vi "JKISM++ State Dashboard - DebugTool.vi"() -> ()   [LabVIEW 2014]
uses:
  _Support/Typedef/_JKISM Current State.ctl
  _Support/GlobalEvent/FGV-GlobalEventRef.vi
  <resource>/dialog/lvconfig.llb/LV Config Write Numeric (I32).vi
  <resource>/dialog/lvconfig.llb/LV Config Read Numeric (I32).vi
  _Support/jkism-tool-support.lvlib
  JKI State Machine++.lvlib
panel:
  in  "Clear JKISM":bool
  out "Dashboard":T1(array[cluster])
  out "State History":string
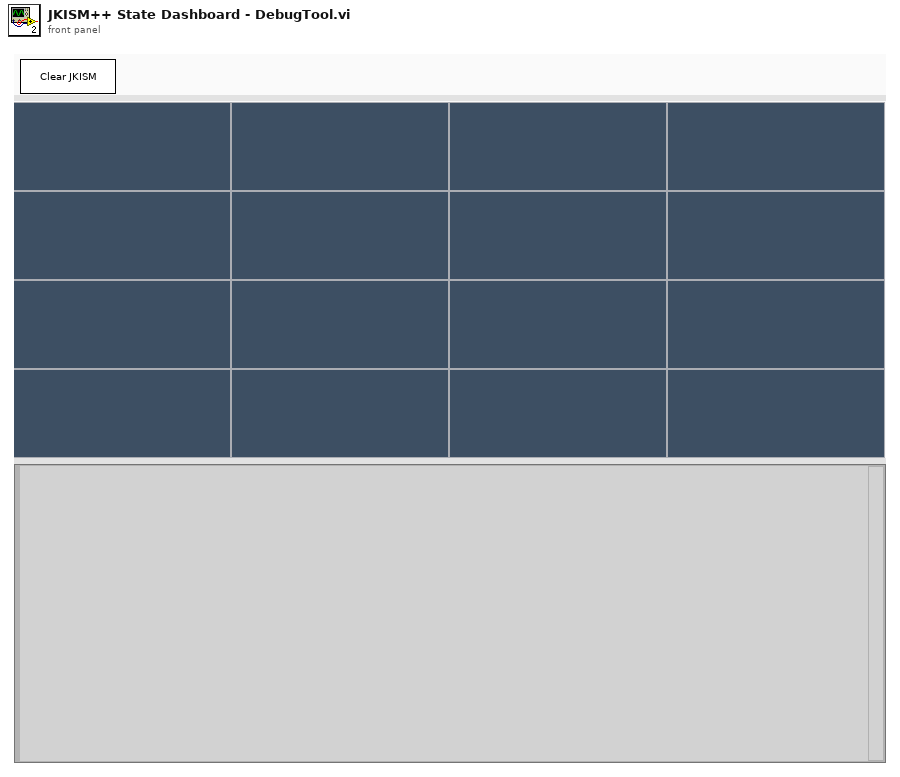
[diagram p1: front panel]
types:
  T1 = cluster{"Label":string, "Value":string, "String":string}[][]
  T2 = enum32{"Invalid", "Standard", "Closed", "Hidden", "Minimized", "Maximized"}
  T3 = enum32{"invalid app kind", "Development System", "Run Time System", "Student Edition", "Embedded LabVIEW", "Evaluation", "Custom"}
  T4 = typedef "JKI State Machine++.lvlib/_JKISM Current State.ctl" = cluster{"Name(\"\" to use uuid)":string, "Current State":string, "Arguments":string, "Argument - State":string, "From Who":string, "Complete(T)/Start(F)":bool}
  T5 = cluster{"Label":string, "Value":string, "String":string}
  T6 = cluster{"Core":cluster{"Current VI Reference":refnum<vi>, "Close Panel on Exit?":bool}, "Global-DataTable":string[][], "NumCols":i16, "NumRows":i16, "JKISM Global Log Event":refnum<user-event>, "Log":T4}
  T7 = cluster{"Current VI Reference":refnum<vi>, "Close Panel on Exit?":bool}
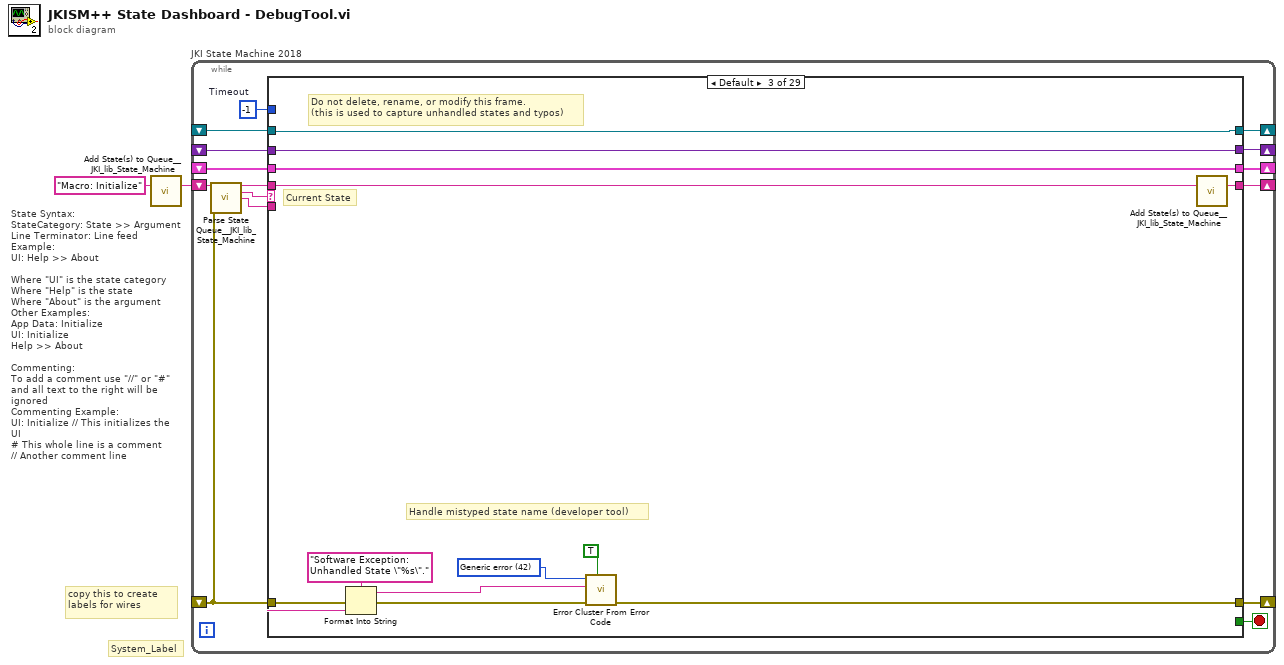
[diagram p0: block diagram]
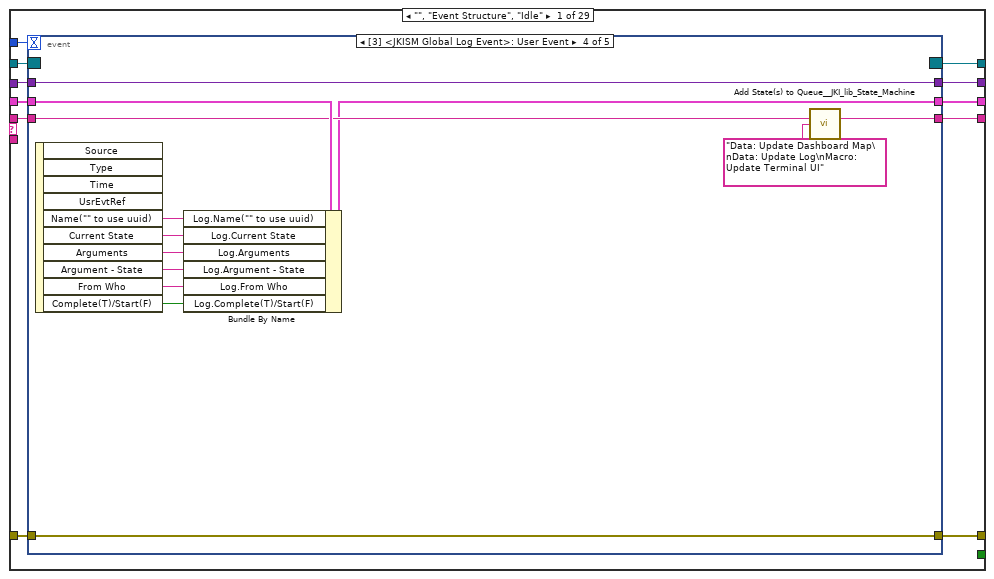
[diagram p2: hidden frame]
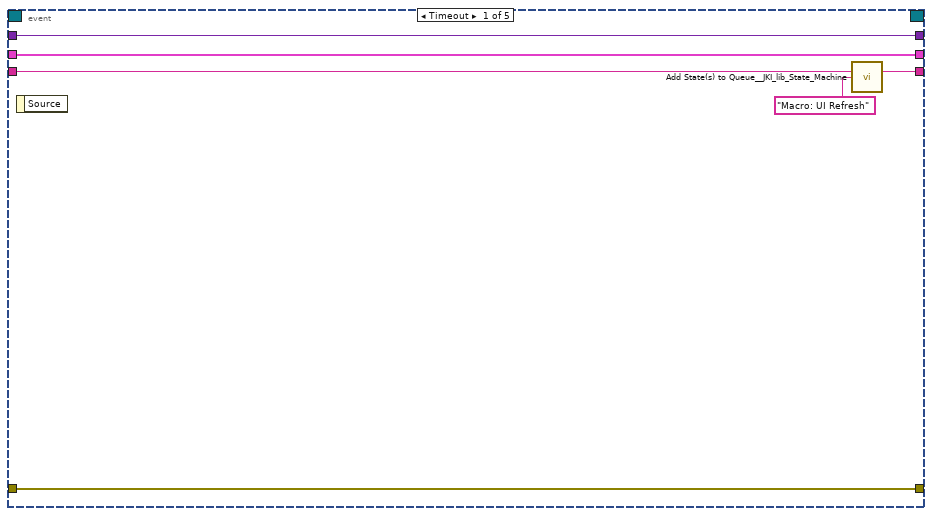
[diagram p3: hidden frame]
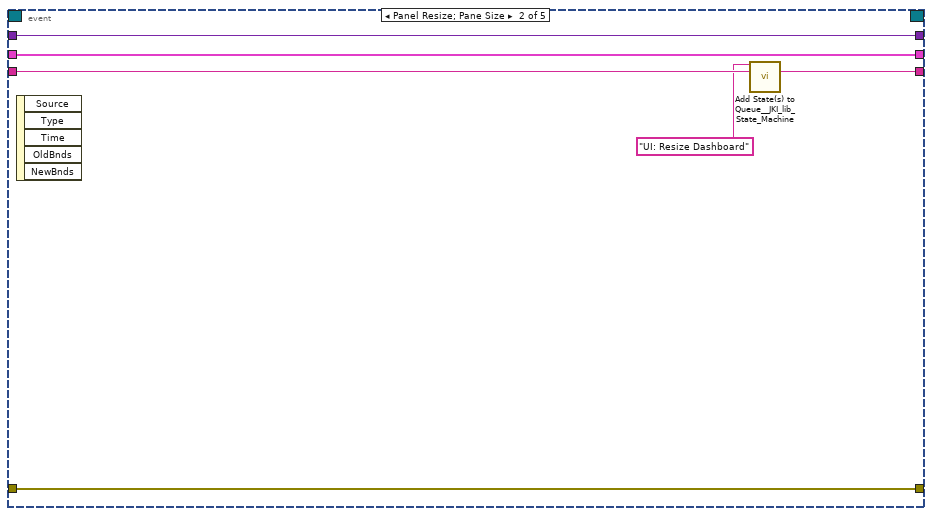
[diagram p4: hidden frame]
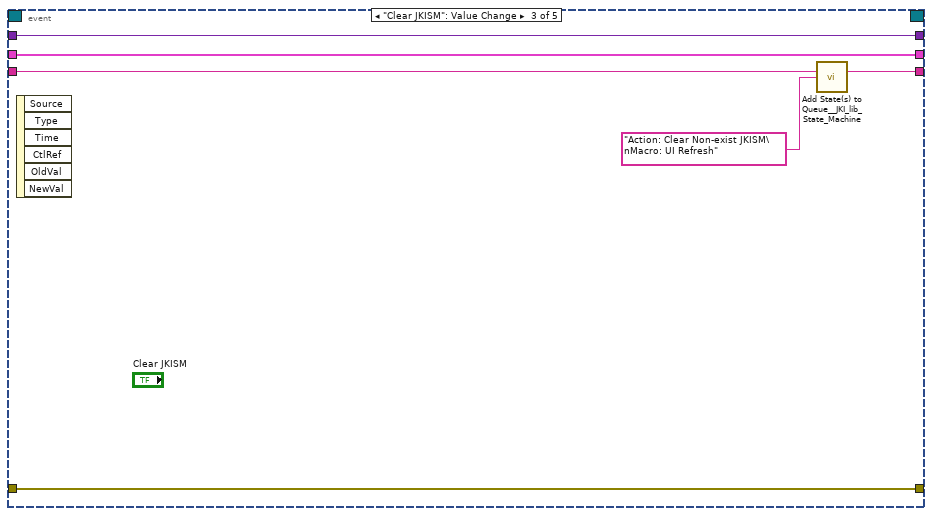
[diagram p5: hidden frame]
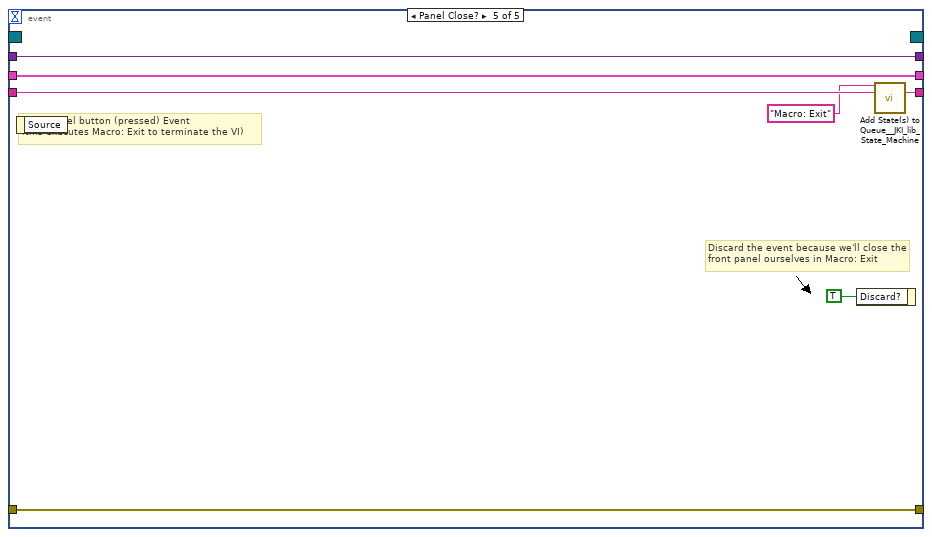
[diagram p6: hidden frame]
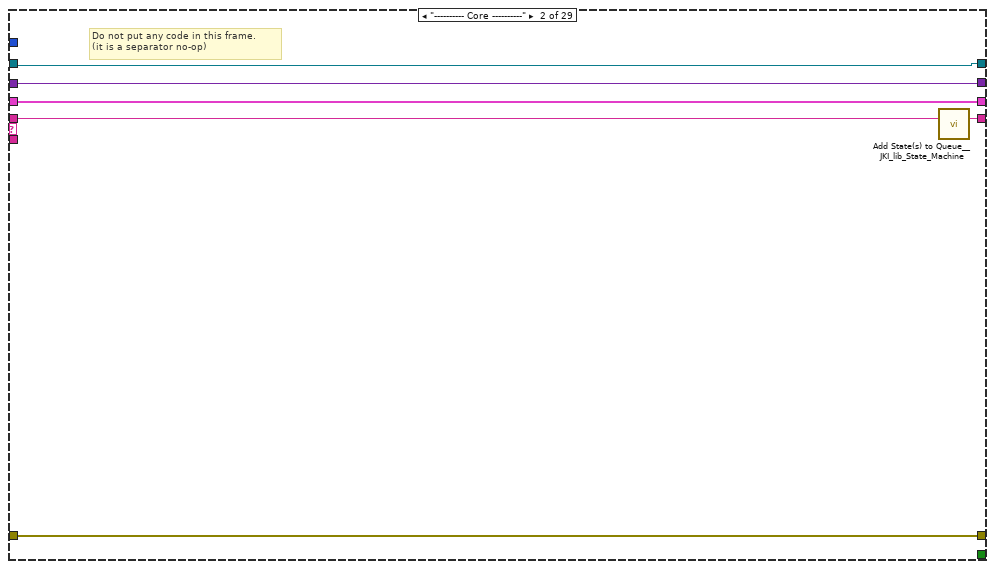
[diagram p7: hidden frame]
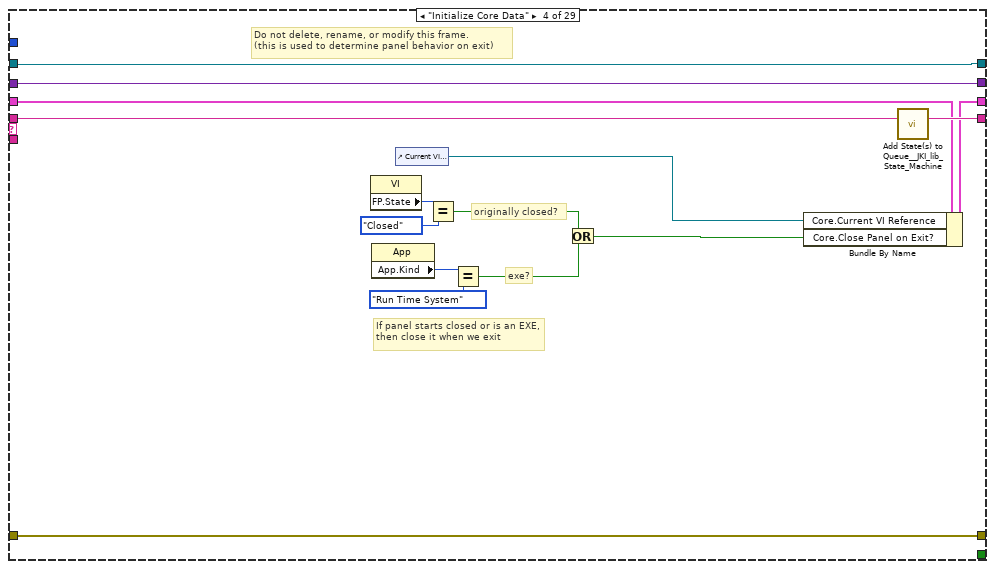
[diagram p8: hidden frame]
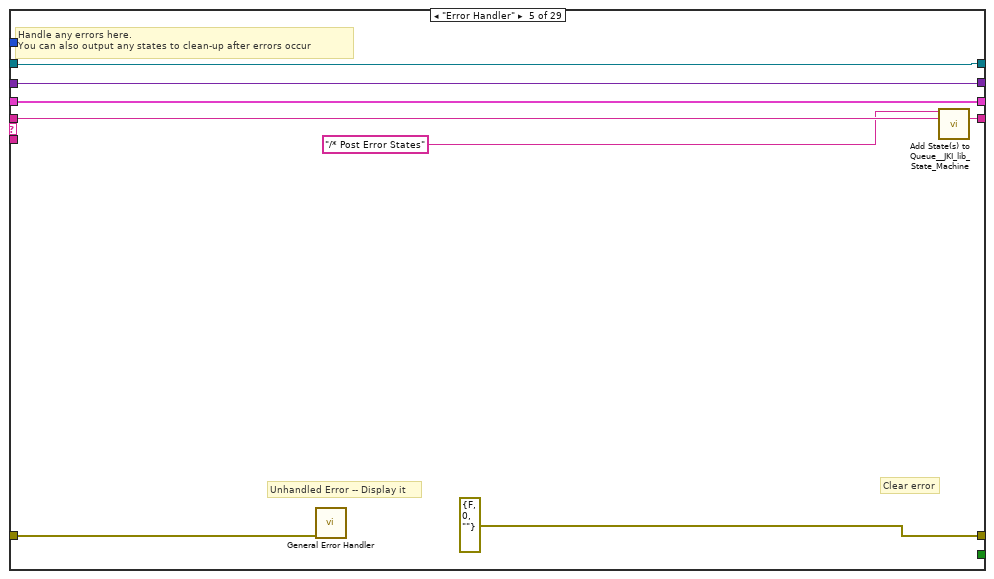
[diagram p9: hidden frame]
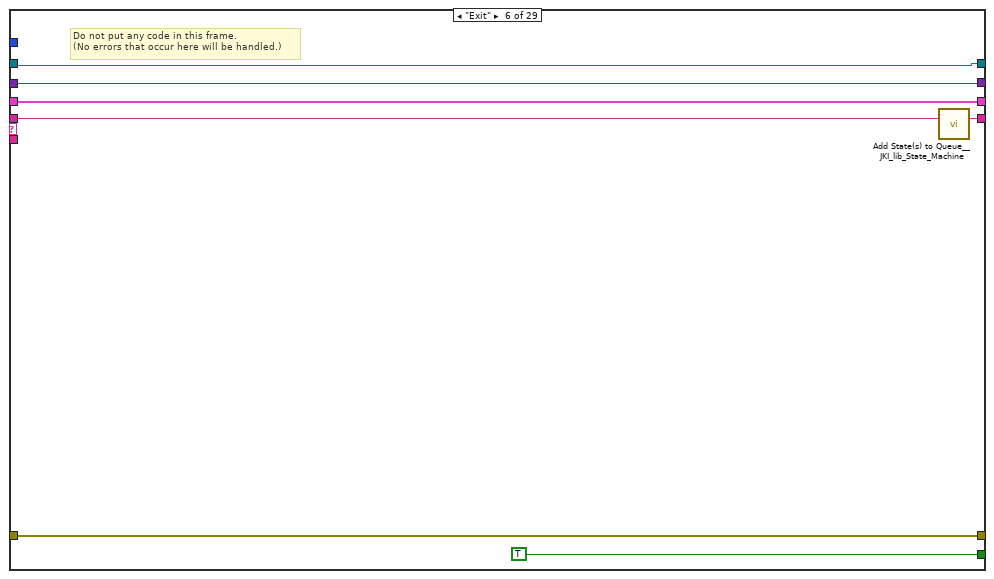
[diagram p10: hidden frame]
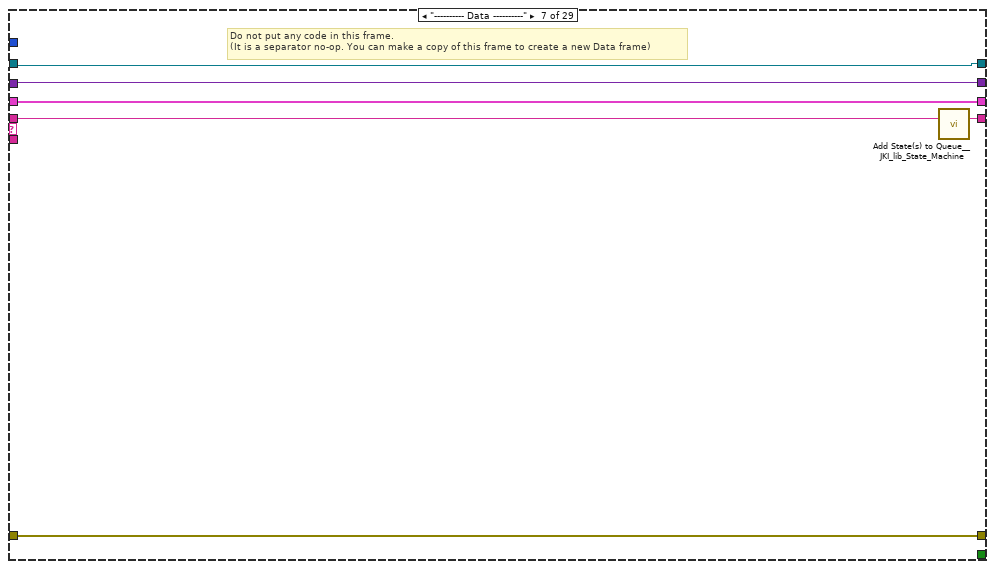
[diagram p11: hidden frame]
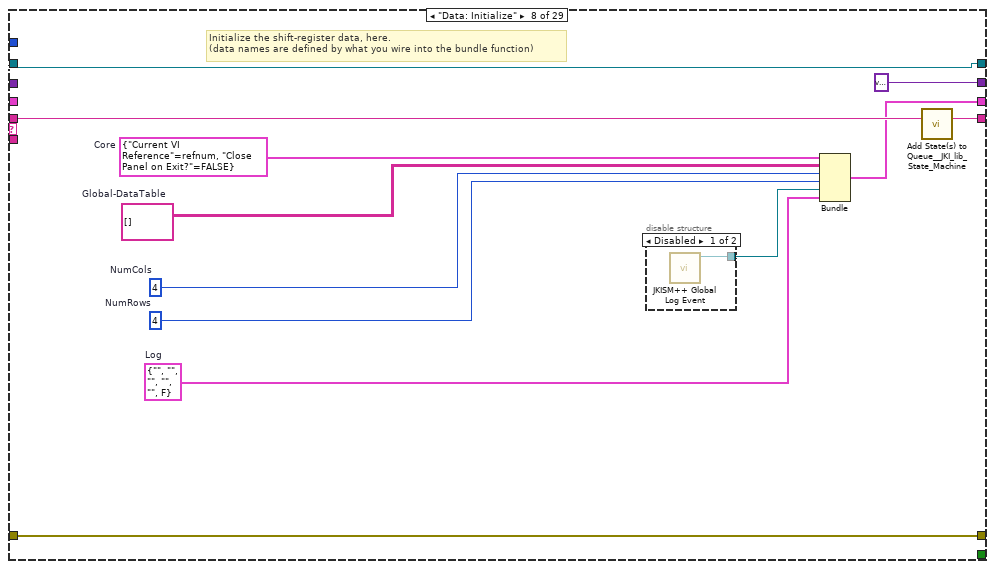
[diagram p12: hidden frame]
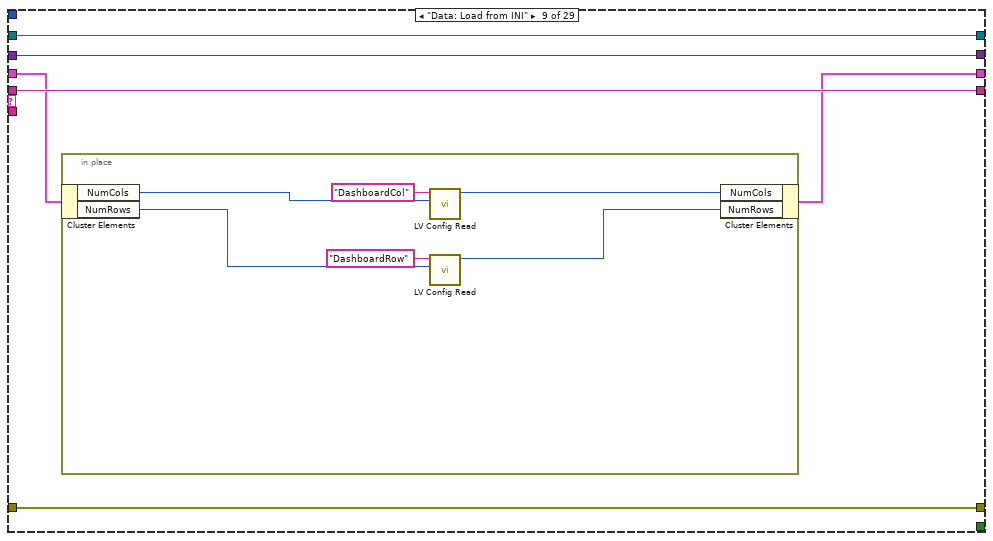
[diagram p14: hidden frame]
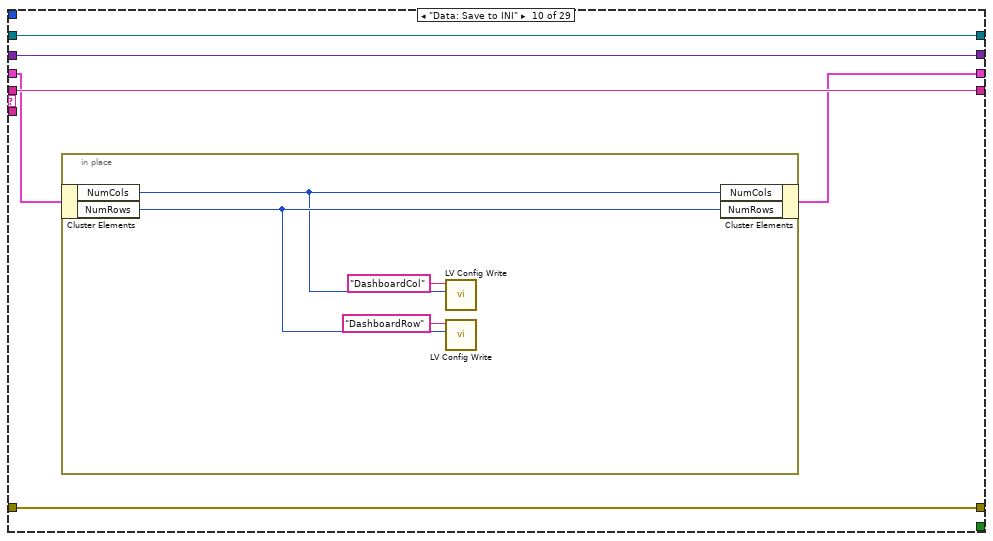
[diagram p15: hidden frame]
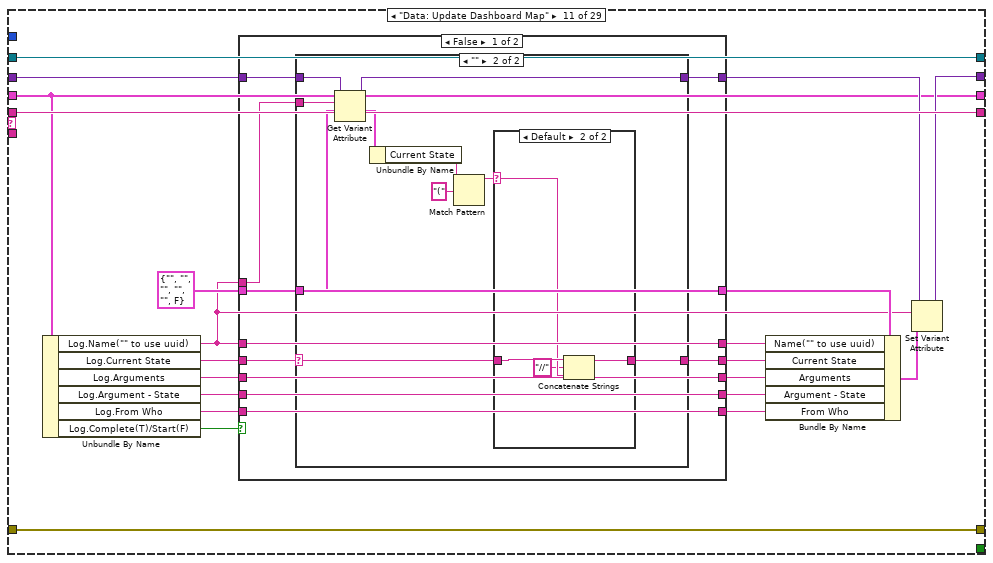
[diagram p16: hidden frame]
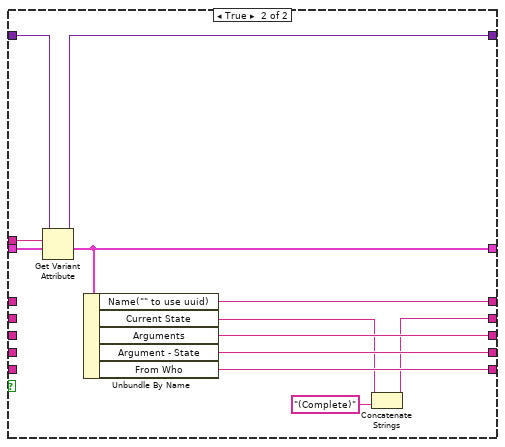
[diagram p19: hidden frame]
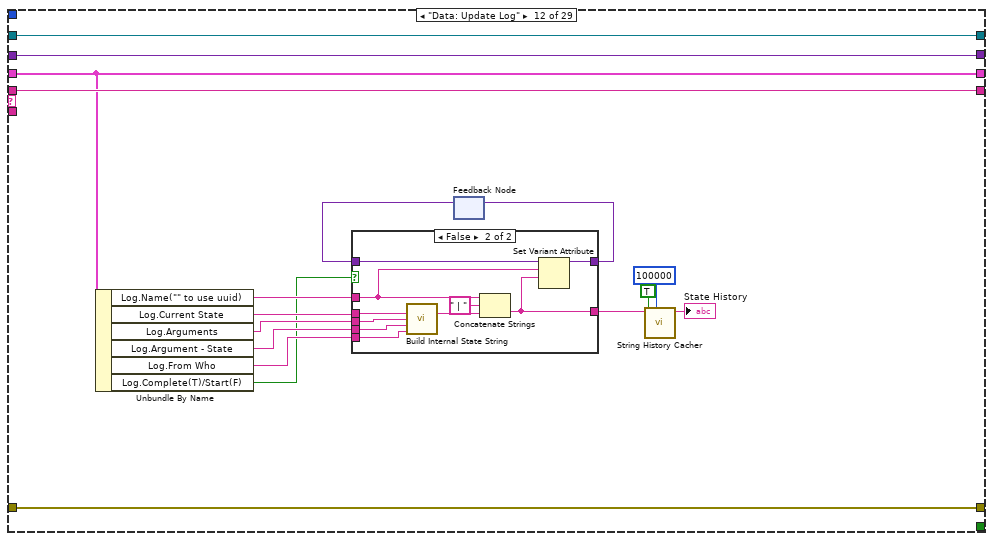
[diagram p20: hidden frame]
diagram:
  # "State Syntax:\nStateCategory: State >> Argument\nLine Terminator: Line feed\nExample:\nUI: Help >> About\n\nWhere \"UI\" is the state category\nWhere \"Help\" is the state\nWhere \"About\" is the argument\nOther Examples:\nApp Data: Initialize\nUI: Initialize\nHelp >> About\n\nCommenting:\nTo add a comment use \"//\" or \"#\" and all text to the right will be ignored\nCommenting Example:\nUI: Initialize // This initializes the UI\n# This whole line is a comment\n// Another comment line"
  # "copy this to create labels for wires"
  # "System_Label"
  n1 = call <vilib>:"Add State(s) to Queue__JKI_lib_State_Machine.vi"("State(s) in (\"\")"="Macro: Initialize") -> ("States Out"=w1:string)  [unwired: 14 in]
  n2 = while "JKI State Machine 2018" {
    shift-right: [w10] -> _
    shift-left: _ -> [w9]
    shift-right: [w13] -> _
    shift-left: _ -> [w7]
    shift-right: [w12] -> _
    shift-left: w1 -> [w14]
    shift-right: [w6] -> _
    shift-left: _ -> [w5]
    shift-right: [w4] -> _
    shift-left: _ -> [w3]
    stop <- w11 stop-if-true
    w8 = -1  # Timeout
    n3 = call <vilib>:"Parse State Queue__JKI_lib_State_Machine.vi"("State Queue"=w14, "Error In (no error)"=w7) -> ("Remaining States"=w16:string, "Current State"=w17:string, "Arguments"=w15:string)  [unwired: 11 in]
    n4 = case shown="Default" w17 {
      selector: w17 -> [_ _ w75 _ _ _ _ _ _ _ _ _ _ _ _ _ _ _ _ _ _ _ _ _ _ _ _ _ _]
      tunnel: w16 -> [w28 w72 w79 w100 w108 w115 w121 w133 w139 w151 w176 w232 w259 w265 w274 w286 w299 w376 w391 w401 w409 w417 w424 w431 w439 w446 w459 w463 w474]
      tunnel: w15 -> [_ _ _ _ _ _ _ _ _ _ _ _ _ _ _ w281 w293 _ _ _ _ _ _ _ _ _ _ _ _]
      tunnel: w9 -> [w26 w69 w77 w93 w105 w113 w118 _ w138 w150 w163 w223 w254 w262 w270 w284 w295 w372 w388 w400 w408 w413 w421 w428 w434 w443 w456 w462 w473]
      tunnel: [w25 w70 w81 w97 errorcluster {"status"=FALSE, "code"=0, "source"=""} ("error out") w112 w119 w129 w140 w152 w177 w233 w253 w263 w272 w282 w296 w373 w389 w402 w410 w418 w422 w429 w437 w444 w457 w464 w475] -> w13
      tunnel: w7 -> [w24 w70 w80 w97 w104 w112 w119 w129 w140 w152 w177 w233 w256 w263 w272 w283 w297 _ w389 w402 w410 w418 w422 w429 w437 w444 w457 w464 w475]
      tunnel: [w27 w71 w78 w99 w107 w114 w120 w132 w139 w151 w176 w232 w258 w264 w273 w285 w298 w375 w390 w401 w409 w417 w423 w430 w438 w445 w458 w463 w474] -> w12
      tunnel: [_ _ _ _ _ TRUE _ _ _ _ _ _ _ _ _ _ _ _ _ _ _ _ _ _ _ _ _ _ _] -> w11
      tunnel: [w23 w69 w77 w98 w105 w113 w118 w131 w137 w149 w163 w223 w254 w262 w270 w284 w295 w372 w388 w400 w404 w413 w421 w428 w434 w443 w456 w462 w473] -> w10
      tunnel: w8 -> [w22 _ _ _ _ _ _ _ _ _ _ _ _ _ _ _ _ _ _ _ _ _ _ _ _ _ _ _ _]
      tunnel: [w20 w68 w74 w87 w102 w110 w117 variant w136 w148 w164 w231 w252 w261 w267 w280 w292 w369 w383 w399 w407 w416 w420 w426 w433 w441 w449 w461 w469] -> w6
      tunnel: w5 -> [w21 w68 w74 w87 w102 w110 w117 _ w136 w148 w165 w231 w252 w261 w267 w280 w292 w369 w382 w399 w407 w416 w420 w426 w433 w441 w449 w461 w471]
      tunnel: [w18 w67 w73 w86 w101 w109 w116 w124 w135 w147 w175 w230 w251 w260 w266 w279 w291 w368 w379 w398 w405 w415 w419 w425 w432 w440 w448 w460 w472] -> w4
      tunnel: w3 -> [w19 w67 w73 w86 w101 w109 w116 w124 w135 w147 w175 w230 w251 w260 w266 w279 w291 w368 w379 w398 _ w415 w419 w425 w432 w440 w448 w460 w472]
      frame "", "Event Structure", "Idle" {
        n5 = event shown="[3] <JKISM Global Log Event>: User Event" {
          selector: w19 -> [_ _ _ _ _]
          dyn-events: [_ _ _ _ _] -> w18
          timeout: w22 -> [_ _ _ _ _]
          tunnel: w28 -> [w34 w37 w43 w54 w66]
          tunnel: [w33 w38 w42 w58 w65] -> w27
          tunnel: w26 -> [w31 w39 w45 w55 w64]
          tunnel: [w32 w40 w46 w59 w61] -> w25
          tunnel: w24 -> [w32 w40 w46 w59 w61]
          tunnel: [w31 w39 w45 w53 w64] -> w23
          tunnel: w21 -> [w29 w35 w44 w56 w60]
          tunnel: [w29 w35 w44 w56 w60] -> w20
          event Timeout {
            n6 = event-data() -> ()  [unwired: 1 in, 1 out]
            n7 = call <vilib>:"Add State(s) to Queue__JKI_lib_State_Machine.vi"("State(s) in (\"\")"=w34, "State(s) at Back (\"\")"="Macro: UI Refresh" ("State(s) in Front (\"\")")) -> ("States Out"=w33:string)  [unwired: 13 in]
          }
          event Panel Resize; Pane Size {
            n8 = event-data() -> ()  [unwired: 1 in, 5 out]
            n9 = call <vilib>:"Add State(s) to Queue__JKI_lib_State_Machine.vi"("State(s) in Front (\"\")"="UI: Resize Dashboard" ("State(s) in Front (\"\")"), "State(s) in (\"\")"=w37) -> ("States Out"=w38:string)  [unwired: 13 in]
          }
          event "Clear JKISM": Value Change {
            n10 = event-data() -> ()  [unwired: 1 in, 6 out]
            n11 = call <vilib>:"Add State(s) to Queue__JKI_lib_State_Machine.vi"("State(s) in (\"\")"=w43, "State(s) at Back (\"\")"="Action: Clear Non-exist JKISM\nMacro: UI Refresh" ("State(s) at Back (\"\")")) -> ("States Out"=w42:string)  [unwired: 13 in]
          }
          event User Event {
            n12 = event-data() -> ("Name(\"\" to use uuid)"=w47:string, "Current State"=w48:string, "Arguments"=w49:string, "Argument - State"=w50:string, "From Who"=w51:string, "Complete(T)/Start(F)"=w52:bool)  [unwired: 1 in, 4 out]
            n13 = Bundle By Name(cluster=w55, "Log.Name(\"\" to use uuid)"=w47, "Log.Current State"=w48, "Log.Arguments"=w49, "Log.Argument - State"=w50, "Log.From Who"=w51, "Log.Complete(T)/Start(F)"=w52) -> (w53:T6)
            n14 = call <vilib>:"Add State(s) to Queue__JKI_lib_State_Machine.vi"("State(s) in (\"\")"=w54, "State(s) at Back (\"\")"="Data: Update Dashboard Map\nData: Update Log\nMacro: Update Terminal UI" ("State(s) at Back (\"\")")) -> ("States Out"=w58:string)  [unwired: 13 in]
          }
          event Panel Close? {
            # "Discard the event because we'll close the front panel ourselves in Macro: Exit"
            # "Close Panel button (pressed) Event\n(this executes Macro: Exit to terminate the VI)"
            n15 = event-data() -> ()  [unwired: 1 in, 1 out]
            n16 = event-data("Discard?"=TRUE) -> ()  [unwired: 1 in, 1 out]
            n17 = call <vilib>:"Add State(s) to Queue__JKI_lib_State_Machine.vi"("State(s) in Front (\"\")"="Macro: Exit", "State(s) in (\"\")"=w66) -> ("States Out"=w65:string)  [unwired: 13 in]
          }
        }
      }
      frame "---------- Core ----------" {
        # "Do not put any code in this frame.\n(it is a separator no-op)"
        n18 = call <vilib>:"Add State(s) to Queue__JKI_lib_State_Machine.vi"("State(s) in (\"\")"=w72) -> ("States Out"=w71:string)  [unwired: 14 in]
      }
      frame Default {
        w84 = 42 items=["No error", "Argument error", "Memory is full", "Out of zone", "End of file", "File already open", "Generic file I/O error", "File not found", "File permission error", "Disk is full", "Duplicate path", "Too many files open", "System feature not enabled", "Resource file not found", "Cannot add resource", "Resource not found", "Image not found", "Image memory error", "Pen does not exist", "Config type invalid", "Config token not found", "Config parse error", "Config memory error", "Bad external code format", "Bad external code offset", "External code not present", "Null window", "Destroy window error", "Null menu", "Print aborted", "Bad print record", "Print driver error", "Windows error during printing", "Memory error during printing", "Print dialog error", "Generic print error", "Invalid device refnum", "Device not found", "Device parameter error", "Device unit error", "Cannot open device", "Device call aborted", "Generic error", "Cancelled by user", "Object ID too low", "Object ID too high", "Object not in heap", "Unknown heap", "Unknown object (invalid DefProc)", "Unknown object (DefProc not in table)", "Message out of range", "Invalid (null) method", "Unknown message", "Manager call not supported", "Bad address", "Network operation in progress", "Network operation timed out", "Connection is busy", "Network attribute not supported", "Network error", "Address in use", "System out of memory", "Connection aborted", "Connection refused", "Not connected", "Already connected", "Connection closed", "Initialization error (interapplication manager)", "Bad occurrence", "Wait on unbound occurrence handler", "Occurrence queue overflow", "Datalog type conflict", "Unused", "Unrecognized type (interapplication manager)", "Memory corrupt", "Failed to make temporary DLL", "Old CIN version", "Drag socket not found", "Failed to load drop-object", "Failed to register OLE object", "Failed to release OLE object", "Format specifier type mismatch", "Unknown format specifier", "Too few format specifiers", "Too many format specifiers", "Scan failed", "Newer CIN version", "Error converting to variant", "Runtime menu error", "Password tampered", "Variant attribute not found", "Incompatible variant data type", "Event data is not available", "Event Store is not present", "Occurrence is not found", "Event Queue is not created", "Event info is not available", "Refnum passed is NULL", "Error retrieving Class GUID", "Error retrieving CoClass GUID", "Error retrieving TypeLib GUID.", "Bad built application magic bytes.", "Specific driver is different from the specific driver associated with the Logical Name.", "There is no session opened to the class driver.", "Max Error", "MAX - Error with config objects", "MAX - Error loading configuration", "MAX - Group not supported"]
        # "Current State"
        # "Do not delete, rename, or modify this frame.\n(this is used to capture unhandled states and typos)"
        # "Handle mistyped state name (developer tool)"
        n19 = Format Into String(format string="Software Exception: Unhandled State \"%s\"." ("message"), error in=w80, w75) -> (resulting string=w83:string, error out=w82:errorcluster)  [unwired: 1 in]
        n20 = call <vilib>:"Error Cluster From Error Code.vi"("show call chain? (False)"=TRUE, "error in (no error)"=w82, "error message (\"\")"=w83, "error code (0)"=w84) -> ("error out"=w81:errorcluster)  [unwired: 5 in]
        n21 = call <vilib>:"Add State(s) to Queue__JKI_lib_State_Machine.vi"("State(s) in (\"\")"=w79) -> ("States Out"=w78:string)  [unwired: 14 in]
      }
      frame "Initialize Core Data" {
        # "Do not delete, rename, or modify this frame.\n(this is used to determine panel behavior on exit)"
        # "originally closed?"
        # "exe?"
        # "If panel starts closed or is an EXE, then close it when we exit"
        n22 = property class="VI"() -> ("FP.State"=w90:T2)  [unwired: 2 in, 2 out]
        n23 = property class="App"() -> ("App.Kind"=w96:T3)  [unwired: 2 in, 2 out]
        n24 = control-ref of="Current VI Reference"() -> (w91:refnum<vi>)
        n25 = Equal?(x=w90, y=T2."Closed" ("Front Panel Window:State")) -> (x = y?=w88:bool)
        n26 = Equal?(x=w96, y=T3."Run Time System" ("Application:Kind")) -> (x = y?=w94:bool)
        n27 = Or(x=w88, y=w94) -> (x .or. y?=w92:bool)
        n28 = Bundle By Name(cluster=w93, "Core.Current VI Reference"=w91, "Core.Close Panel on Exit?"=w92) -> (w98:T6)
        n29 = call <vilib>:"Add State(s) to Queue__JKI_lib_State_Machine.vi"("State(s) in (\"\")"=w100) -> ("States Out"=w99:string)  [unwired: 14 in]
      }
      frame "Error Handler" {
        # "Unhandled Error -- Display it"
        # "Handle any errors here.\nYou can also output any states to clean-up after errors occur"
        # "Clear error"
        n30 = call <vilib>:"General Error Handler.vi"("error in (no error)"=w104) -> ()  [unwired: 10 in, 5 out]
        n31 = call <vilib>:"Add State(s) to Queue__JKI_lib_State_Machine.vi"("State(s) in Front (\"\")"="/* Post Error States", "State(s) in (\"\")"=w108) -> ("States Out"=w107:string)  [unwired: 13 in]
      }
      frame "Exit" {
        # "Do not put any code in this frame.\n(No errors that occur here will be handled.)"
        n32 = call <vilib>:"Add State(s) to Queue__JKI_lib_State_Machine.vi"("State(s) in (\"\")"=w115) -> ("States Out"=w114:string)  [unwired: 14 in]
      }
      frame "---------- Data ----------" {
        # "Do not put any code in this frame.\n(It is a separator no-op. You can make a copy of this frame to create a new Data frame)"
        n33 = call <vilib>:"Add State(s) to Queue__JKI_lib_State_Machine.vi"("State(s) in (\"\")"=w121) -> ("States Out"=w120:string)  [unwired: 14 in]
      }
      frame "Data: Initialize" {
        w122 = T4 {"Name(\"\" to use uuid)"="", "Current State"="", "Arguments"="", "Argument - State"="", "From Who"="", "Complete(T)/Start(F)"=FALSE}  # Log
        w127 = i16 4  # NumCols
        w126 = i16 4  # NumRows
        w128 = string[][] []  # Global-DataTable
        w130 = T7 {"Current VI Reference"=refnum, "Close Panel on Exit?"=FALSE}  # Core
        # "Initialize the shift-register data, here.\n(data names are defined by what you wire into the bundle function)"
        n34 = disable-structure shown="Disabled" {
          disable-tunnel: [w134 _] -> w123
          frame Disabled {
            n35 = call "JKISM++ Global Log Event.vi"() -> ("JKISM Global Log Event"=w134:refnum<user-event>)  [unwired: 10 in, 1 out]
          }
          frame Enabled {
          }
        }
        n36 = Bundle("Core"=w130, "Global-DataTable"=w128, "NumCols"=w127, "NumRows"=w126, "JKISM Global Log Event"=w123, "Log"=w122) -> (w131:T6)  [unwired: 1 in]
        n37 = call <vilib>:"Add State(s) to Queue__JKI_lib_State_Machine.vi"("State(s) in (\"\")"=w133) -> ("States Out"=w132:string)  [unwired: 14 in]
      }
      frame "Data: Load from INI" {
        n38 = in-place {
          n39 = in-place-cluster #1(w138) -> ("NumCols"=w142:i16, "NumRows"=w145:i16)
          n40 = call-poly <resource>:"LV Config Read.vi"("default value"=w142, "key"="DashboardCol") -> ("value"=w141:i32)  [unwired: 3 in, 2 out]
          n41 = call-poly <resource>:"LV Config Read.vi"("default value"=w145, "key"="DashboardRow") -> ("value"=w144:i32)  [unwired: 3 in, 2 out]
          n42 = in-place-cluster #1("NumCols"=w141, "NumRows"=w144) -> (w137:T6)
        }
      }
      frame "Data: Save to INI" {
        n43 = in-place {
          n44 = in-place-cluster #2(w150) -> ("NumCols"=w153:i16, "NumRows"=w154:i16)
          n45 = call-poly <resource>:"LV Config Write.vi"("value"=w153, "key"="DashboardCol") -> ()  [unwired: 5 in, 1 out]
          n46 = call-poly <resource>:"LV Config Write.vi"("value"=w154, "key"="DashboardRow") -> ()  [unwired: 5 in, 1 out]
          n47 = in-place-cluster #2("NumCols"=w153, "NumRows"=w154) -> (w149:T6)
        }
      }
      frame "Data: Update Dashboard Map" {
        n48 = Unbundle By Name(w163) -> ("Log.Name(\"\" to use uuid)"=w157:string, "Log.Current State"=w162:string, "Log.Arguments"=w161:string, "Log.Argument - State"=w160:string, "Log.From Who"=w159:string, "Log.Complete(T)/Start(F)"=w158:bool)
        n49 = case shown="False" w158 {
          tunnel: w165 -> [w183 w216]
          tunnel: [w182 w215] -> w173
          tunnel: T4 {"Name(\"\" to use uuid)"="", "Current State"="", "Arguments"="", "Argument - State"="", "From Who"="", "Complete(T)/Start(F)"=FALSE} ("Cross JKI State Machine Data") -> [w180 w214]
          tunnel: w157 -> [w181 w213]
          tunnel: w159 -> [w187 _]
          tunnel: [w187 w212] -> w171
          tunnel: w160 -> [w186 _]
          tunnel: [w186 w211] -> w170
          tunnel: w161 -> [w185 _]
          tunnel: [w185 w210] -> w169
          tunnel: w162 -> [w179 _]
          tunnel: [w178 w205] -> w168
          tunnel: w157 -> [w184 _]
          tunnel: [w184 w207] -> w167
          tunnel: [w180 w208] -> w166
          frame False {
            n50 = case shown="\"\"" w179 {
              selector: w179 -> [w188 w191]
              tunnel: w183 -> [w189 w199]
              tunnel: [w189 w198] -> w182
              tunnel: w181 -> [_ w197]
              tunnel: w180 -> [_ w195]
              tunnel: [w188 w190] -> w178
              frame Default {
              }
              frame "" {
                n51 = Get Variant Attribute(Variant=w199, name=w197, default value (empty Variant)=w195) -> (duplicate Variant=w198:variant, value=w196:T4)  [unwired: 1 in, 2 out]
                n52 = Unbundle By Name(w196) -> ("Current State"=w194:string)
                n53 = Match Pattern(string=w194, regular expression="(") -> (before substring=w192:string)  [unwired: 1 in, 3 out]
                n54 = case shown="Default" w192 {
                  selector: w192 -> [_ w202]
                  tunnel: w191 -> [w200 w204]
                  tunnel: [w200 w203] -> w190
                  frame "" {
                  }
                  frame Default {
                    n55 = Concatenate Strings(w204, "//" ("string"), w202) -> (w203:string)
                  }
                }
              }
            }
          }
          frame True {
            n56 = Get Variant Attribute(Variant=w216, name=w213, default value (empty Variant)=w214) -> (duplicate Variant=w215:variant, value=w208:T4)  [unwired: 1 in, 2 out]
            n57 = Unbundle By Name(w208) -> ("Name(\"\" to use uuid)"=w207:string, "Current State"=w206:string, "Arguments"=w210:string, "Argument - State"=w211:string, "From Who"=w212:string)
            n58 = Concatenate Strings(w206, "(Complete)" ("string")) -> (w205:string)
          }
        }
        n59 = Bundle By Name(cluster=w166, "Name(\"\" to use uuid)"=w167, "Current State"=w168, "Arguments"=w169, "Argument - State"=w170, "From Who"=w171) -> (w174:T4)
        n60 = Set Variant Attribute(Variant=w173, name=w157, value=w174) -> (Variant out=w164:variant)  [unwired: 1 in, 2 out]
      }
      frame "Data: Update Log" {
        n61 = Unbundle By Name(w223) -> ("Log.Name(\"\" to use uuid)"=w222:string, "Log.Current State"=w221:string, "Log.Arguments"=w220:string, "Log.Argument - State"=w219:string, "Log.From Who"=w218:string, "Log.Complete(T)/Start(F)"=w217:bool)
        n62 = feedback #3() -> (w226:variant)  [unwired: 1 in]
        n63 = case shown="False" w217 {
          tunnel: w221 -> [_ w249]
          tunnel: w220 -> [_ w248]
          tunnel: w219 -> [_ w247]
          tunnel: w218 -> [_ w246]
          tunnel: w226 -> [w240 w244]
          tunnel: [w239 w243] -> w225
          tunnel: w222 -> [w238 w242]
          tunnel: [w236 w241] -> w224
          frame True {
            n64 = Get Variant Attribute(Variant=w240, name=w238, default value (empty Variant)="") -> (duplicate Variant=w239:variant, value=w235:string)  [unwired: 1 in, 2 out]
            n65 = Concatenate Strings(w235, "(Complete)" ("string")) -> (w236:string)
          }
          frame False {
            n66 = call "Build Internal State String.vi"("State"=w249, "Arguments (\"\")"=w248, "Arg-State (\"\")"=w247, "Source (\"\")"=w246) -> ("State with Arguments"=w250:string)  [unwired: 11 in]
            n67 = Concatenate Strings(w242, " | " ("string"), w250) -> (w241:string)
            n68 = Set Variant Attribute(Variant=w244, name=w242, value=w241) -> (Variant out=w243:variant)  [unwired: 1 in, 2 out]
          }
        }
        n69 = feedback-in #3(w225) -> ()
        n70 = call "String History Cacher.vi"("length"=100000, "Include Timestamp(F)"=TRUE, "String"=w224) -> ("String Cache"=→"State History":string)  [unwired: 8 in]
      }
      frame "Data: Cleanup" {
        # "Cleanup any data and references, here.\n(this is called automatically, by the Macro: Exit)"
        n71 = Unbundle By Name(w254) -> ("Core.Current VI Reference"=w257:refnum<vi>)
        n72 = Close Reference(reference=w257, error in (no error)=w256) -> (error out=w255:errorcluster)
        n73 = Merge Errors(w255) -> (w253:errorcluster)
        n74 = call <vilib>:"Add State(s) to Queue__JKI_lib_State_Machine.vi"("State(s) in (\"\")"=w259) -> ("States Out"=w258:string)  [unwired: 14 in]
      }
      frame "---------- UI ----------" {
        # "Do not put any code in this frame.\n(It is a separator no-op. You can make a copy of this frame to create a new UI frame)"
        n75 = call <vilib>:"Add State(s) to Queue__JKI_lib_State_Machine.vi"("State(s) in (\"\")"=w265) -> ("States Out"=w264:string)  [unwired: 14 in]
      }
      frame "UI: Initialize" {
        # "Initialize the User Interface, here.\n(this is called automatically, by the Macro: Init)"
        n76 = invoke class="VI" method="Default Vals.Reinit All"() -> (error out=w271:errorcluster)  [unwired: 3 in, 2 out]
        n77 = Unbundle By Name(w270) -> ("NumRows"=w269:i16, "NumCols"=w268:i16)
        n78 = flat-sequence {
          tunnel: w271 -> [_]
          tunnel: w269 -> [w276]
          tunnel: w268 -> [w275]
          frame #0 {
            n79 = Initialize Array(T5 {"Label"="", "Value"="", "String"=""} ("Dashboard"), w276, w275) -> (w277:T1)
            n80 = local write "Dashboard"(w277) -> ()
          }
        }
        n81 = call <vilib>:"Add State(s) to Queue__JKI_lib_State_Machine.vi"("State(s) in (\"\")"=w274) -> ("States Out"=w273:string)  [unwired: 14 in]
      }
      frame "UI: Cursor Set" {
        # "Argument"
        # "Set and Unset Cursor Busy.\n(Usage: \"UI: Cursor Set >> Busy|Idle\")"
        n82 = case shown="\"Idle\", Default" w281 {
          tunnel: w283 -> [w288 w290]
          tunnel: [w287 w289] -> w282
          frame "Idle", Default {
            n83 = call <vilib>:"Unset Busy.vi"("error in (no error)"=w288) -> ("error out"=w287:errorcluster)  [unwired: 10 in]
          }
          frame "Busy" {
            n84 = call <vilib>:"Set Busy.vi"("error in (no error)"=w290) -> ("error out"=w289:errorcluster)  [unwired: 9 in, 1 out]
          }
        }
        n85 = call <vilib>:"Add State(s) to Queue__JKI_lib_State_Machine.vi"("State(s) in (\"\")"=w286) -> ("States Out"=w285:string)  [unwired: 14 in]
      }
      frame "UI: Front Panel State" {
        # "Argument"
        # "Set Front Panel Open or Closed\n(Usage: \"UI: Front Panel State >> Open|Close\")"
        n86 = Unbundle By Name(w295) -> ("Core.Current VI Reference"=w294:refnum<vi>)
        n87 = case shown="\"Minimize\", \"Minimized\"" w293 {
          tunnel: w297 -> [w305 w320 w331 w344 w357]
          tunnel: [w307 w321 w333 w346 w359] -> w296
          tunnel: w294 -> [w306 w318 w332 w345 w358]
          frame "Open", "Standard", Default {
            w300 = T2."Standard" ("State")
            n88 = property class="VI"(reference=w306, error in=w305) -> (reference out=w303:refnum<vi>, error out=w304:errorcluster, "FP.State"=w302:T2)
            n89 = Not Equal?(x=w302, y=w300) -> (x != y?=w301:bool)
            n90 = case shown="True" w301 {
              tunnel: [w311 w313] -> w307
              tunnel: w304 -> [w310 w313]
              tunnel: w303 -> [w309 _]
              tunnel: w300 -> [w308 _]
              frame True {
                n91 = invoke class="VI" method="FP.Open"(reference=w309, error in=w310, "Activate"=TRUE, "State"=w308) -> (error out=w311:errorcluster)  [unwired: 1 in, 4 out]
              }
              frame False {
              }
            }
          }
          frame "Close", "Closed" {
            n92 = property class="VI"(reference=w318, error in=w320) -> (reference out=w317:refnum<vi>, error out=w319:errorcluster, "FP.State"=w315:T2)
            n93 = Not Equal?(x=w315, y=T2."Closed" ("Front Panel Window:State")) -> (x != y?=w314:bool)
            n94 = case shown="True" w314 {
              tunnel: [w322 w325] -> w321
              tunnel: w319 -> [w322 w324]
              tunnel: w317 -> [_ w323]
              frame False {
              }
              frame True {
                n95 = invoke class="VI" method="FP.Close"(reference=w323, error in=w324) -> (error out=w325:errorcluster)  [unwired: 1 in, 2 out]
              }
            }
          }
          frame "Hidden", "Hide" {
            w326 = T2."Hidden" ("State")
            n96 = property class="VI"(reference=w332, error in=w331) -> (reference out=w329:refnum<vi>, error out=w330:errorcluster, "FP.State"=w328:T2)
            n97 = Not Equal?(x=w328, y=w326) -> (x != y?=w327:bool)
            n98 = case shown="True" w327 {
              tunnel: [w337 w338] -> w333
              tunnel: w330 -> [w336 w338]
              tunnel: w329 -> [w335 _]
              tunnel: w326 -> [w334 _]
              frame True {
                n99 = invoke class="VI" method="FP.Open"(reference=w335, error in=w336, "State"=w334) -> (error out=w337:errorcluster)  [unwired: 2 in, 4 out]
              }
              frame False {
              }
            }
          }
          frame "Minimize", "Minimized" {
            w339 = T2."Minimized" ("State")
            n100 = property class="VI"(reference=w345, error in=w344) -> (reference out=w342:refnum<vi>, error out=w343:errorcluster, "FP.State"=w341:T2)
            n101 = Not Equal?(x=w341, y=w339) -> (x != y?=w340:bool)
            n102 = case shown="True" w340 {
              tunnel: [w350 w351] -> w346
              tunnel: w343 -> [w349 w351]
              tunnel: w342 -> [w348 _]
              tunnel: w339 -> [w347 _]
              frame True {
                n103 = invoke class="VI" method="FP.Open"(reference=w348, error in=w349, "State"=w347) -> (error out=w350:errorcluster)  [unwired: 2 in, 4 out]
              }
              frame False {
              }
            }
          }
          frame "Maximize", "Maximized" {
            w352 = T2."Maximized" ("State")
            n104 = property class="VI"(reference=w358, error in=w357) -> (reference out=w355:refnum<vi>, error out=w356:errorcluster, "FP.State"=w354:T2)
            n105 = Not Equal?(x=w354, y=w352) -> (x != y?=w353:bool)
            n106 = case shown="True" w353 {
              tunnel: [w363 w364] -> w359
              tunnel: w356 -> [w362 w364]
              tunnel: w355 -> [w361 _]
              tunnel: w352 -> [w360 _]
              frame True {
                n107 = invoke class="VI" method="FP.Open"(reference=w361, error in=w362, "State"=w360) -> (error out=w363:errorcluster)  [unwired: 2 in, 4 out]
              }
              frame False {
              }
            }
          }
        }
        n108 = call <vilib>:"Add State(s) to Queue__JKI_lib_State_Machine.vi"("State(s) in (\"\")"=w299) -> ("States Out"=w298:string)  [unwired: 14 in]
      }
      frame "UI: Resize Dashboard" {
        # "Do not put any code in this frame.\n(It is a separator no-op. You can make a copy of this frame to create a new UI frame)"
        n109 = control-ref of="Pane 3"() -> (w367:refnum<vi>)
        n110 = property class="Pane"(reference=w367) -> ("Width"=w366:u32, "Height"=w365:u32)  [unwired: 1 in, 2 out]
        n111 = control-ref of="Dashboard"() -> (w374:refnum<vi>)
        n112 = Unbundle By Name(w372) -> ("NumCols"=w370:i16, "NumRows"=w371:i16)
        n113 = call "Dashboard Cell2 Array Resize.vi"("Num Columns"=w370, "Num Rows"=w371, "area height"=w365, "area width"=w366, "Array 2"=w374) -> ("error out"=w373:errorcluster)  [unwired: 6 in]
        n114 = call <vilib>:"Add State(s) to Queue__JKI_lib_State_Machine.vi"("State(s) in (\"\")"=w376) -> ("States Out"=w375:string)  [unwired: 14 in]
      }
      frame "UI: Update Dashboard" {
        # "Do not put any code in this frame.\n(It is a separator no-op. You can make a copy of this frame to create a new UI frame)"
        n115 = Get Variant Attribute(Variant=w382) -> (duplicate Variant=w383:variant, names=w381:string[], values=w380:variant[])  [unwired: 3 in, 1 out]
        n116 = Variant To Data(type=T4[] [], Variant=w380) -> (data=w377:T4[])  [unwired: 1 in, 1 out]
        n117 = for {
          tunnel: w381 -> [w396] mode=indexing
          tunnel: [w395] -> w387 mode=indexing
          tunnel: w377 -> [w394] mode=indexing
          n118 = Unbundle By Name(w394) -> ("Current State"=w393:string, "Arguments"=w392:string)  [unwired: 1 out]
          n119 = Bundle By Name(cluster=T5 {"Label"="", "Value"="", "String"=""}, "Label"=w396, "Value"=w393, "String"=w392) -> (w395:T5)
        }
        n120 = Unbundle By Name(w388) -> ("NumRows"=w385:i16, "NumCols"=w384:i16)
        n121 = Reshape Array(w387, w385, w384) -> (→"Dashboard":T1)
        n122 = call <vilib>:"Add State(s) to Queue__JKI_lib_State_Machine.vi"("State(s) in (\"\")"=w391) -> ("States Out"=w390:string)  [unwired: 14 in]
      }
      frame "--------- Event ---------" {
      }
      frame "Register User Event" {
        n123 = call "JKISM++ Global Log Event.vi"() -> ("Error out"=w406:errorcluster, "JKISM Global Log Event"=w403:refnum<user-event>)  [unwired: 10 in]
        n124 = register-events(error in=w406, w403) -> (reference out=w405:refnum<event-registration>)  [unwired: 1 in, 1 out]
        n125 = Bundle By Name(cluster=w408, "JKISM Global Log Event"=w403) -> (w404:T6)
      }
      frame "UnRegister User Event" {
        n126 = Unregister For Events(event registration refnum=w415) -> (error out=w414:errorcluster)  [unwired: 1 in]
        n127 = Unbundle By Name(w413) -> ("JKISM Global Log Event"=w412:refnum<user-event>)
        n128 = call "JKISM++ Destroy Global Log Event.vi"("Error in"=w414, "JKISM Global Log Event"=w412) -> ("Error out"=w411:errorcluster)  [unwired: 9 in]
        n129 = call <vilib>:"Clear Errors.vi"("error in (no error)"=w411) -> ()  [unwired: 6 in, 1 out]
      }
      frame "---------- Macro ----------" {
        # "Do not put any code in this frame.\n(It is a separator no-op. You can make a copy of this frame to create a new Macro frame)"
        n130 = call <vilib>:"Add State(s) to Queue__JKI_lib_State_Machine.vi"("State(s) in (\"\")"=w424) -> ("States Out"=w423:string)  [unwired: 14 in]
      }
      frame "Macro: Initialize" {
        # "Initialization Macro\n(This is called once, when the VI starts)"
        n131 = call <vilib>:"Add State(s) to Queue__JKI_lib_State_Machine.vi"("State(s) in Front (\"\")"="Data: Initialize\nInitialize Core Data\nData: Load from INI\nUI: Initialize\nUI: Resize Dashboard\nRegister User Event\n//UI: Front Panel State >> Open", "State(s) in (\"\")"=w431) -> ("States Out"=w430:string)  [unwired: 13 in]
      }
      frame "Macro: UI Refresh" {
        # "Do not put any code in this frame.\n(It is a separator no-op. You can make a copy of this frame to create a new Macro frame)"
        n132 = call <vilib>:"Add State(s) to Queue__JKI_lib_State_Machine.vi"("State(s) at Back (\"\")"="Macro: Update Terminal UI" ("State(s) in Front (\"\")")) -> ("States Out"=w436:string)  [unwired: 14 in]
        n133 = call <vilib>:"Add State(s) to Queue__JKI_lib_State_Machine.vi"("State(s) in Front (\"\")"=w436, "State(s) in (\"\")"=w439) -> ("States Out"=w438:string)  [unwired: 13 in]
      }
      frame "Macro: Update Terminal UI" {
        # "Do not put any code in this frame.\n(It is a separator no-op. You can make a copy of this frame to create a new Macro frame)"
        n134 = call <vilib>:"Add State(s) to Queue__JKI_lib_State_Machine.vi"("State(s) in Front (\"\")"="UI: Update Dashboard" ("State(s) in Front (\"\")"), "State(s) in (\"\")"=w446) -> ("States Out"=w445:string)  [unwired: 13 in]
      }
      frame "Macro: Exit" {
        # "Exit Macro\n(This is called once, when the VI exits)"
        n135 = Unbundle By Name(w456) -> ("Core.Close Panel on Exit?"=w455:bool)
        n136 = Select(t="UI: Front Panel State >> Close", s=w455, f="") -> (s? t:f=w451:string)
        n137 = call <vilib>:"Add State(s) to Queue__JKI_lib_State_Machine.vi"("State(s) in Front (\"\")"="UnRegister User Event" ("State(s) in Front (\"\")"), "State(s) in (\"\")"=w451, "State(s) at Back (\"\")"="Data: Save to INI\nData: Cleanup\nExit") -> ("States Out"=w454:string)  [unwired: 12 in]
        n138 = call <vilib>:"Add State(s) to Queue__JKI_lib_State_Machine.vi"("State(s) in Front (\"\")"=w454, "State(s) in (\"\")"=w459) -> ("States Out"=w458:string)  [unwired: 13 in]
      }
      frame "----- Action ------" {
      }
      frame "Action: Clear Non-exist JKISM" {
        n139 = Get Variant Attribute(Variant=w471) -> (duplicate Variant=w470:variant, names=w468:string[], values=w467:variant[])  [unwired: 3 in, 1 out]
        n140 = Variant To Data(type=T4[] [], Variant=w467) -> (data=w466:T4[])  [unwired: 1 in, 1 out]
        n141 = for {
          shift-right: [w487] -> w469
          shift-left: w470 -> [w488]
          tunnel: w468 -> [w486] mode=indexing
          tunnel: w466 -> [w485] mode=indexing
          n142 = Unbundle By Name(w485) -> ("Current State"=w483:string, "Name(\"\" to use uuid)"=w482:string)
          n143 = Search 1D Array(1D array=string[] ["<Remaining States>", "Exit"], element=w483) -> (index of element=w479:i32)  [unwired: 1 in]
          n144 = Match Pattern(string=w482, regular expression="^-") -> (offset past match=w480:i32)  [unwired: 1 in, 3 out]
          n145 = Greater Or Equal To 0?(x=w479) -> (x >= 0?=w477:bool)
          n146 = Greater Or Equal To 0?(x=w480) -> (x >= 0?=w478:bool)
          n147 = Or(x=w478, y=w477) -> (x .or. y?=w476:bool)
          n148 = case shown="False" w476 {
            tunnel: w488 -> [w489 w492]
            tunnel: [w489 w491] -> w487
            tunnel: w486 -> [_ w490]
            tunnel: w482 -> [_ _]
            tunnel: w483 -> [_ _]
            frame False {
            }
            frame True {
              n149 = Delete Variant Attribute(6:w490, 7:w492) -> (3:w491:variant)  [unwired: 1 in, 2 out]
            }
          }
        }
      }
    }
  }
